vi "Custom Types in Meta Data.vi"() -> ()   [LabVIEW 2017, in "Tree API.lvlib" / "Tree.lvclass"]
uses:
  Tree.lvclass
  API/Set Attribute Tree Data.vi
  Tree Data/Tree Data.lvclass
  Data Types/Bool/To Bool Tree Data.vi
  Data Types/Bool/Bool.lvclass
  Data Types/Error Cluster/Error Cluster.lvclass
  API/Get Attribute Tree Data.vi
  Data Types/Bool/From Bool Tree Data.vi
  Data Types/Int/From Integer Tree Data.vi
  Data Types/Int/Int.lvclass
panel:
  in  "Tab Control":T1(tab)
  in  "Input Error Cluster":errorcluster={"status"=TRUE, "code"=123, "source"="Some description."}
  out "Extracted From Meta Data":errorcluster={"status"=TRUE, "code"=123, "source"="Some description."}
  out "Extracted From Error Cluster TD Type":errorcluster={"status"=TRUE, "code"=123, "source"="Some description."}
  out "Error Status":bool=TRUE
  in  "Tree":string(tree)
  out "XML String":string="<Parent>\n\n<Child>\n<Attr Name=\"Custom Error Type\" Type=\"Bool\" MetaData=\"<Cluster>\r\n<Name>Input Error Cluster</Name>\r\n<NumElts>3</NumElts>\r\n<Boolean>\r\n<Name>status</Name>\r\n<Val>1</Val>\r\n</Boolean>\r\n<I32>\r\n<Name>code</Name>\r\n<Val>123</Val>\r\n</I32>\r\n<String>\r\n<Name>source</Name>\r\n<Val>Some description.</Val>\r\n</String>\r\n</Cluster>\r\n\">TRUE</Attr>\r\n<Attr Name=\"Error Cluster Type\" Type=\"Error Cluster\" >TRUE, 123</Attr>\n\n</Child>\n</Parent>"
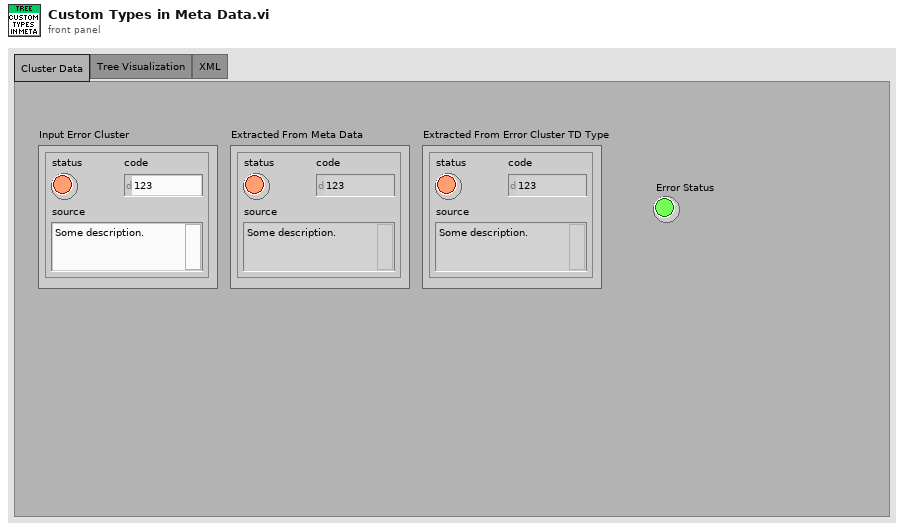
[diagram p1: front panel]
types:
  T1 = enum32{"Cluster Data", "Tree Visualization", "XML"}
  T2 = cluster{"Left Cell String":string, "Child Text":string[], "Child Tag":string, "Item Indent":i32, "Child Only?":bool, "Glyph Index":i32}[]
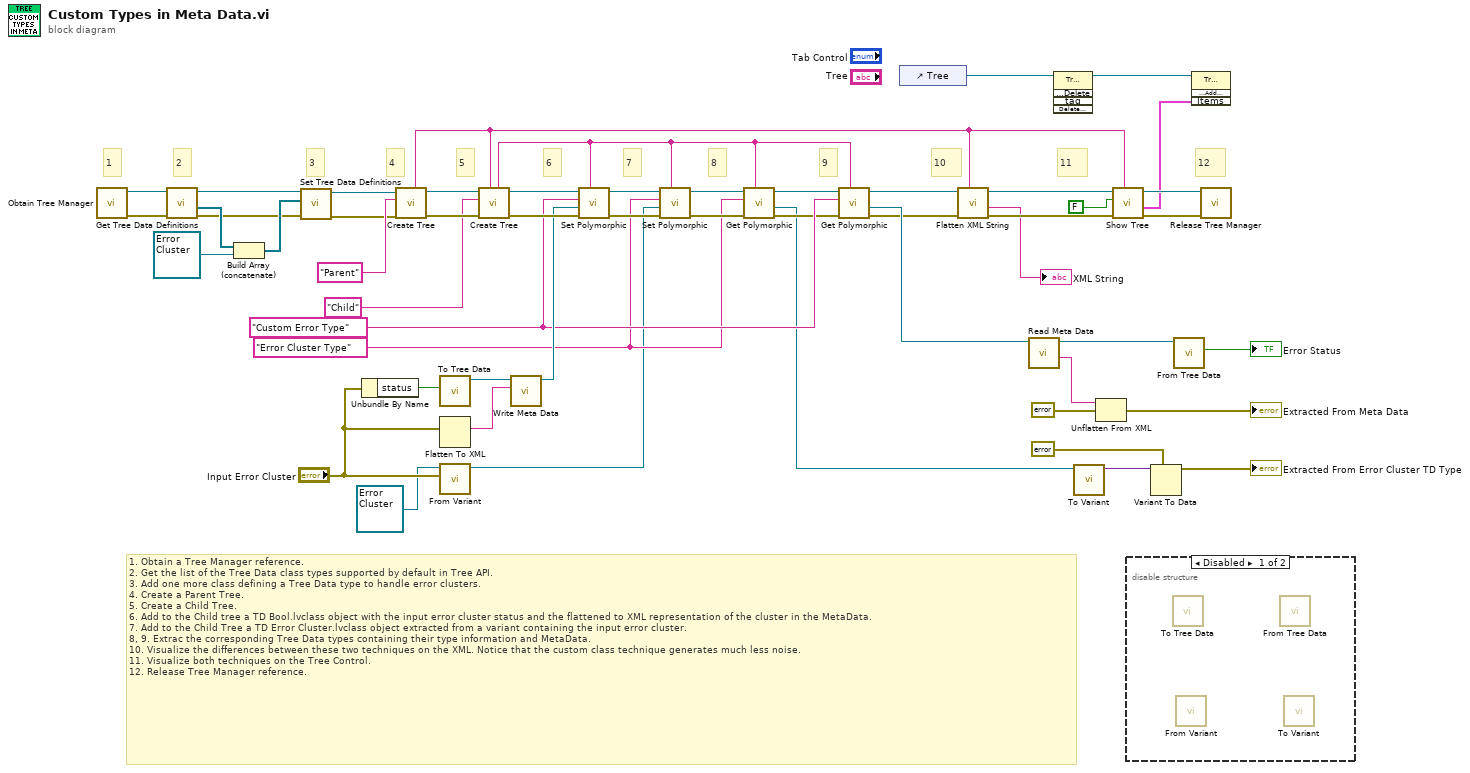
[diagram p0: block diagram]
diagram:
  w28 = "Error Cluster Type" ("Name")
  w43 = "Custom Error Type" ("Name")
  # "1. Obtain a Tree Manager reference.\n2. Get the list of the Tree Data class types supported by default in Tree API.\n3. Add one more class defining a Tree Data type to handle error clusters.\n4. Create a Parent Tree.\n5. Create a Child Tree.\n6. Add to the Child tree a TD Bool.lvclass object with the input error cluster status and the flattened to XML representation of the cluster in the MetaData.\n7. Add to the Child Tree a TD Error Cluster.lvclass object extracted from a variant containing the input error cluster.\n8, 9. Extrac the corresponding Tree Data types containing their type information and MetaData.\n10. Visualize the differences between these two techniques on the XML. Notice that the custom class technique generates much less noise.\n11. Visualize both techniques on the Tree Control.\n12. Release Tree Manager reference."
  # "12"
  # "11"
  # "10"
  # "9"
  # "8"
  # "7"
  # "6"
  # "5"
  # "4"
  # "3"
  # "2"
  # "1"
  n1 = call "Obtain Tree Manager.vi"() -> ("Error Out"=w20:errorcluster, "Tree"=w21:refnum<data-value>)  [unwired: 10 in]
  n2 = call "Get Tree Data Definitions.vi"("Error In"=w20, "Tree Manager"=w21) -> ("Error Out"=w15:errorcluster, "Tree Data Defs"=w18:refnum<class "Tree Data.lvclass">[], "Tree Manager"=w19:refnum<data-value>)  [unwired: 7 in]
  n3 = Build Array (concatenate)(w18, refnum<class "Error Cluster.lvclass"> refnum ("TD Error Cluster.lvclass")) -> (w16:refnum<class "Tree Data.lvclass">[])
  n4 = call "Set Tree Data Definitions.vi"("Error In"=w15, "Tree Data Defs"=w16, "Tree Manager"=w19) -> ("Error Out"=w14:errorcluster, "Tree Manager"=w13:refnum<data-value>)  [unwired: 7 in]
  n5 = Unbundle By Name("Input Error Cluster") -> ("status"=w40:bool)
  n6 = call "Create Tree.vi"("Error In"=w14, "Name"="Parent", "Tree Manager"=w13) -> ("Error Out"=w52:errorcluster, "Tree Manager"=w53:refnum<data-value>, "Unique ID"=w11:string)  [unwired: 6 in]
  n7 = call-poly "To Tree Data.vi"("Boolean"=w40) -> ("Bool Tree Data"=w44:refnum<class "Bool.lvclass">)  [unwired: 10 in]
  n8 = Flatten To XML(anything="Input Error Cluster") -> (xml string=w39:string)
  n9 = call "From Variant.vi"("Variant"="Input Error Cluster", "Tree Data Type"=refnum<class "Error Cluster.lvclass"> refnum ("TD Error Cluster.lvclass")) -> ("Tree Data Out"=w23:refnum<class "Tree Data.lvclass">)  [unwired: 8 in, 1 out]
  n10 = call "Create Tree.vi"("Parent ID (empty)"=w11, "Error In"=w52, "Name"="Child", "Tree Manager"=w53) -> ("Error Out"=w48:errorcluster, "Tree Manager"=w49:refnum<data-value>, "Unique ID"=w31:string)  [unwired: 5 in]
  n11 = call "Write Meta Data.vi"("Meta Data"=w39, "Tree Data In"=w44) -> ("Tree Data Out"=w47:refnum<class "Bool.lvclass">)  [unwired: 9 in]
  n12 = call-poly "Set Polymorphic.vi"("Tree ID"=w31, "Error In"=w48, "Attribute Value"=w47, "Attribute Name"=w43, "Tree Manager"=w49) -> ("Error Out"=w34:errorcluster, "Tree Manager"=w35:refnum<data-value>)  [unwired: 4 in, 1 out]
  n13 = call-poly "Set Polymorphic.vi"("Tree ID"=w31, "Error In"=w34, "Attribute Value"=w23, "Attribute Name"=w28, "Tree Manager"=w35) -> ("Error Out"=w32:errorcluster, "Tree Manager"=w33:refnum<data-value>)  [unwired: 4 in, 1 out]
  n14 = call-poly "Get Polymorphic.vi"("Tree ID"=w31, "Error In"=w32, "Attribute Name"=w28, "Tree Manager"=w33) -> ("Error Out"=w29:errorcluster, "Attribute Value"=w27:refnum<class "Tree Data.lvclass">, "Tree Manager"=w30:refnum<data-value>)  [unwired: 4 in, 1 out]
  n15 = call-poly "Get Polymorphic.vi"("Tree ID"=w31, "Error In"=w29, "Attribute Name"=w43, "Tree Manager"=w30) -> ("Error Out"=w10:errorcluster, "Attribute Value"=w42:refnum<class "Tree Data.lvclass">, "Tree Manager"=w12:refnum<data-value>)  [unwired: 4 in, 1 out]
  n16 = control-ref of="Tree"() -> (w2:refnum<vi>)
  n17 = call "Flatten XML String.vi"("Root ID"=w11, "Error In"=w10, "Tree"=w12) -> ("Error Out"=w8:errorcluster, "XML String"=→"XML String":string, "Tree"=w9:refnum<data-value>)  [unwired: 6 in]
  n18 = call "Read Meta Data.vi"("Tree Data In"=w42) -> ("Meta Data"=w36:string, "Tree Data Out"=w41:refnum<class "Tree Data.lvclass">)  [unwired: 9 in]
  n19 = invoke class="Tree (strict)" method="Edit Tree Items.Delete"(reference=w2) -> (reference out=w3:refnum<vi>)  [unwired: 4 in, 4 out]
  n20 = call "To Variant.vi"("Tree Data"=w27) -> ("Variant"=w26:variant)  [unwired: 9 in, 1 out]
  n21 = Unflatten From XML(xml string=w36, type=errorcluster {"status"=FALSE, "code"=0, "source"=""} ("error in (no error)")) -> (value=→"Extracted From Meta Data":errorcluster)  [unwired: 1 in, 1 out]
  n22 = call "Show Tree.vi"("Root ID"=w11, "Error In"=w8, "Show IDs (False)"=FALSE ("Show IDs (True)"), "Tree"=w9) -> ("Error Out"=w45:errorcluster, "Items Out"=w1:T2, "Tree"=w46:refnum<data-value>)  [unwired: 5 in]
  n23 = disable-structure shown="Disabled" {
    frame Disabled {
      n24 = call-poly "To Tree Data.vi"() -> ()  [unwired: 11 in, 1 out]
      n25 = call "From Variant.vi"() -> ()  [unwired: 10 in, 2 out]
      n26 = call-poly "From Tree Data.vi"() -> ()  [unwired: 11 in, 1 out]
      n27 = call "To Variant.vi"() -> ()  [unwired: 10 in, 2 out]
    }
    frame Enabled {
    }
  }
  n28 = Variant To Data(type=errorcluster {"status"=FALSE, "code"=0, "source"=""} ("error in (no error)"), Variant=w26) -> (data=→"Extracted From Error Cluster TD Type":errorcluster)  [unwired: 1 in, 1 out]
  n29 = call-poly "From Tree Data.vi"("Tree Data"=w41) -> ("Boolean"=→"Error Status":bool)  [unwired: 10 in]
  n30 = invoke class="Tree (strict)" method="Edit Tree Items.Add Multiple Items to End"(reference=w3, "Items"=w1) -> ()  [unwired: 2 in, 4 out]
  n31 = call "Release Tree Manager.vi"("Error In"=w45, "Tree"=w46) -> ()  [unwired: 9 in, 1 out]
